vi "edit tag by name.vi"(8 "error in":errorcluster, 10 "name":string, 11 "engine configuration in":refnum<class "engine configuration.lvclass">) -> (0 "error out":errorcluster, 1 "change?":bool, 3 "engine configuration out":refnum<class "engine configuration.lvclass">)   [LabVIEW 2013, in "PL Framework Configuration Tool.lvlib" / "EngineTags.lvclass"]
uses:
  EngineTags.lvclass
  <vilib>/NI/Module Execution Interface/Engine Configuration/engine configuration.lvclass
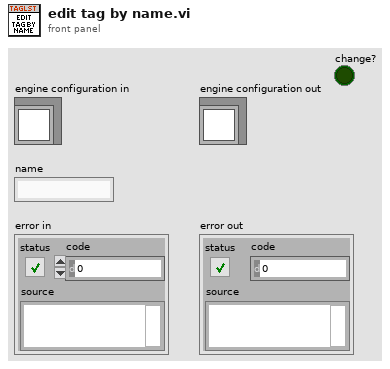
[diagram p1: front panel]
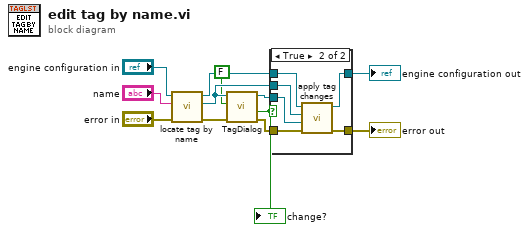
[diagram p0: block diagram]
diagram:
  n1 = call <vilib>:"locate tag by name.vi"("error in"="error in", "tag name"="name", "engine configuration in"="engine configuration in") -> ("error out"=w3:errorcluster, "tag descriptor"=w9:refnum<class "tag descriptor.lvclass">, "engine configuration out"=w6:refnum<class "engine configuration.lvclass">)  [unwired: 6 in]
  n2 = call "TagDialog.vi"("error in"=w3, "new?"=FALSE, "tag"=w9) -> ("error out"=w11:errorcluster, "change?"=w5:bool, "new tag"=w8:refnum<class "tag descriptor.lvclass">)  [unwired: 5 in, 1 out]
  "change?" <- w5
  n3 = case shown="True" w5 {
    tunnel: [w14 w20] -> w7
    tunnel: w6 -> [w14 w19]
    tunnel: w8 -> [_ w18]
    tunnel: w9 -> [_ w17]
    tunnel: w11 -> [w13 w16]
    tunnel: [w13 w15] -> w12
    frame False {
    }
    frame True {
      n4 = call <vilib>:"apply tag changes.vi"("error in"=w16, "modified tag"=w18, "original tag"=w17, "engine configuration in"=w19) -> ("error out"=w15:errorcluster, "engine configuration out"=w20:refnum<class "engine configuration.lvclass">)  [unwired: 6 in]
    }
  }
  "error out" <- w12
  "engine configuration out" <- w7
